vi "Vision Processing.vi"(7 "CameraDevRef":T1) -> ()   [LabVIEW 2011]
doc: "This VI runs in parallel to other tasks. It gets images from the camera, processes them for color or shape and use that information to affect robot behavior."
uses:
  <vilib>/Rock Robotics/WPI/Camera/WPI_CameraDevRef.ctl
  Robot Global Data.vi
  <vilib>/vision/NI_Vision_Development_Module.lvlib
panel:
  in  "Case to run":dbl=2.0
  in  "Manual Overide":bool
  out "Target Distance":dbl
  out "Target Y Coord":dbl
  out "Distance Array":dbl[](array[numeric])
  in  "Scaler":dbl=0.85
  in  "Enable Imaging on Screen":bool
  out "Target X Coord":dbl
  in  "Lower Speed Limit":dbl=0.05
  out "Turret Rotation":dbl
  out "Number of Rectangles Visible":dbl
  out "Y Position Array":dbl[](array[numeric])
  out "X Position Array":dbl[](array[numeric])
  out "Array":T2(array[cluster])
  in  "Score Limits":T3={"Rect Coverage"=76.0, "Aspect Ratio"=40.0, "X Edge Strength"=40.0, "Y Edge Strength"=60.0}
  out "Processed Image":T4(plugin-control)
  out "Original Image":T4(plugin-control)
  in  "Annotate":bool=TRUE
  in  "Particle Count Limit":i32=10
  in  "Area Size Limit":i32=444
  in  "Range":cluster{"Lower value":sgl, "Upper value":sgl}={"Lower value"=120.0, "Upper value"=255.0}
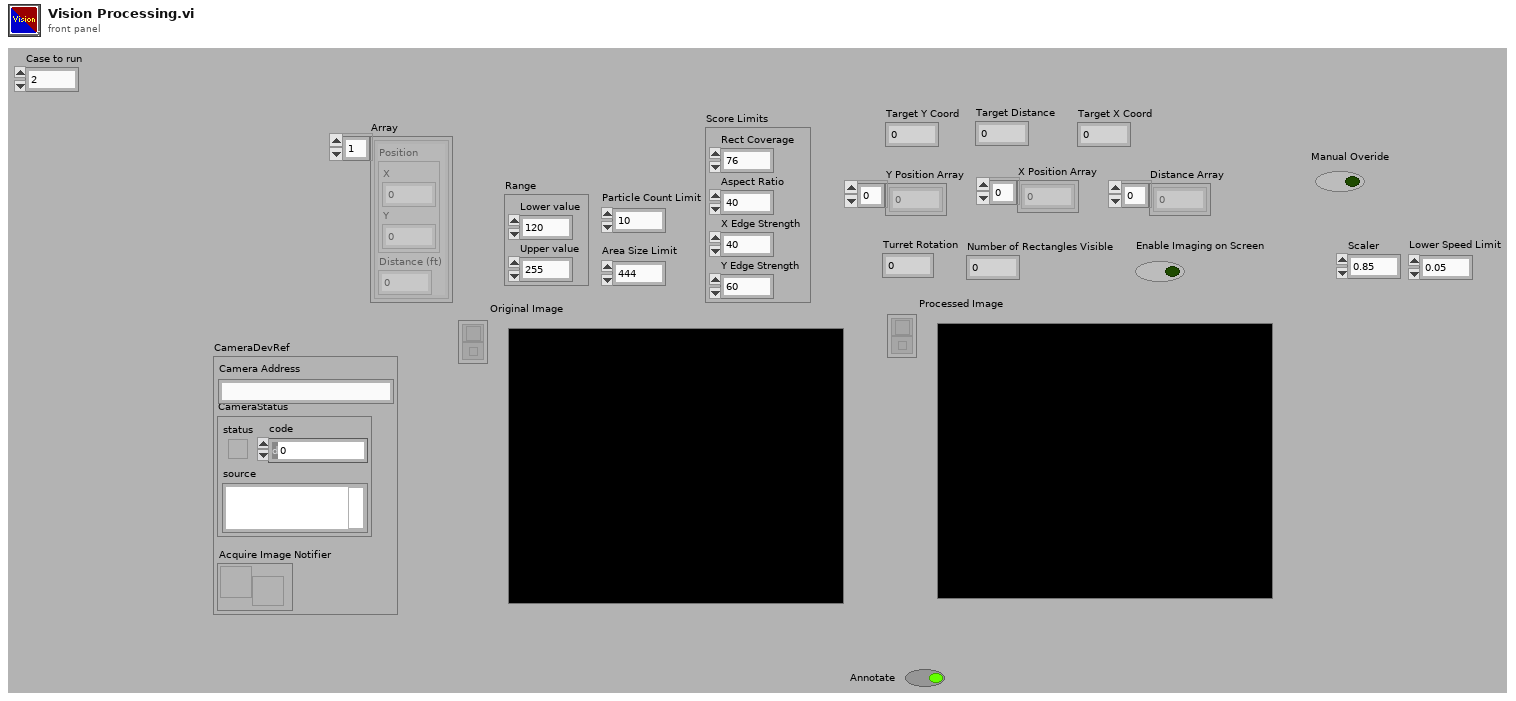
[diagram p1: front panel]
types:
  T1 = typedef "WPI_CameraDevRef.ctl" = cluster{"Camera Address":string, "CameraStatus":errorcluster, "Acquire Image Notifier":refnum<notifier>}
  T2 = cluster{"Position":cluster{"X":dbl, "Y":dbl}, "Distance (ft)":dbl}[]
  T3 = cluster{"Rect Coverage":dbl, "Aspect Ratio":dbl, "X Edge Strength":dbl, "Y Edge Strength":dbl}
  T4 = typedef "IMAQ Image.ctl" = refnum<image>
  T5 = typedef "Image Type" = u32
  T6 = cluster{cluster{"Left":dbl, "Top":dbl, "Right":dbl, "Bottom":dbl}, dbl[]}[]
  T7 = cluster{"Left":dbl, "Top":dbl, "Right":dbl, "Bottom":dbl}
  T8 = cluster{"Target Center (-1 to 1)":cluster{"X":dbl, "Y":dbl}, "Distance (ft)":dbl}
  T9 = cluster{"Target Center (-1 to 1)":cluster{"X":dbl, "Y":dbl}, "Distance (ft)":dbl}[]
  T10 = cluster{"Axis 1":dbl, "Axis 2":dbl, "Axis 3":dbl, "Axis 4":dbl, "Axis 5":dbl, "Axis 6":dbl, "Button 1":bool, "Button 2":bool, "Button 3":bool, "Button 4":bool, "Button 5":bool, "Button 6":bool, "Button 7":bool, "Button 8":bool, "Button 9":bool, "Button 10":bool, "Button 11":bool, "Button 12":bool}
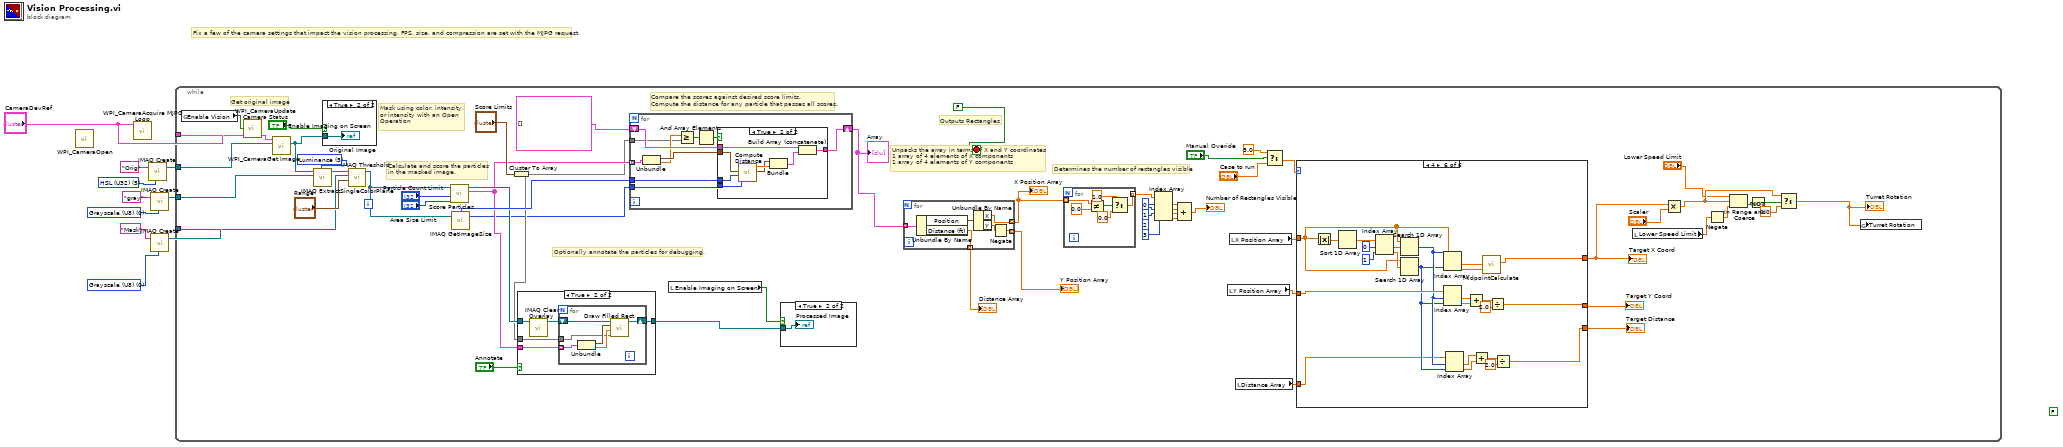
[diagram p0: block diagram]
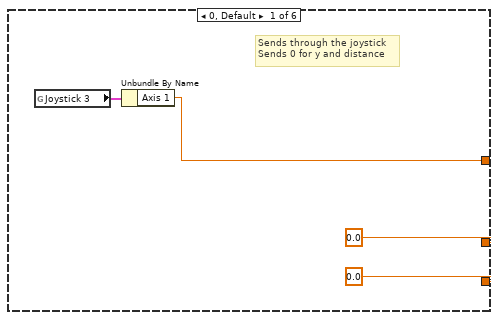
[diagram p4: hidden frame]
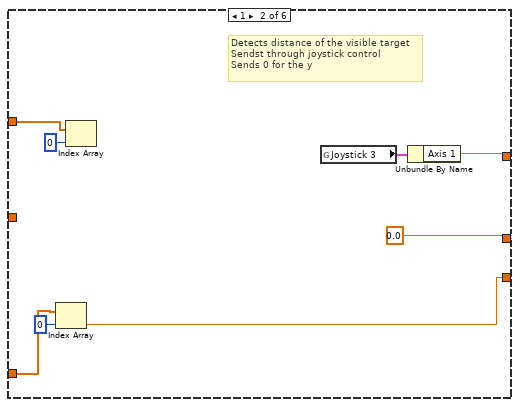
[diagram p5: hidden frame]
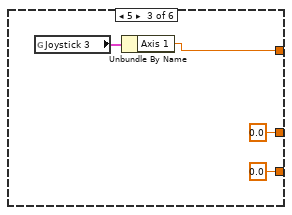
[diagram p6: hidden frame]
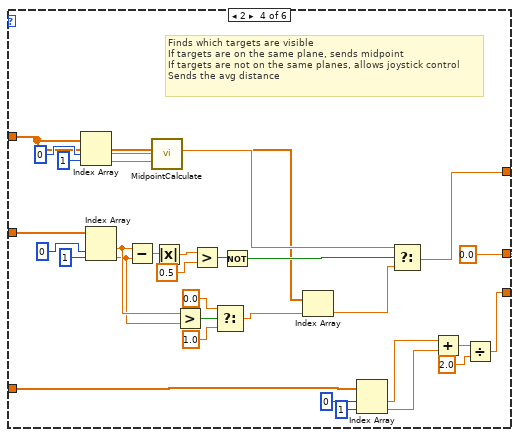
[diagram p7: hidden frame]
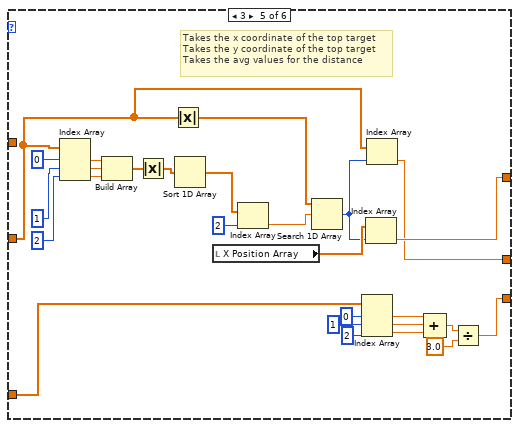
[diagram p8: hidden frame]
diagram:
  w3 = T5 5 items=["Grayscale (U8)", "Grayscale (I16)", "Grayscale (SGL)", "Complex (CSG)", "RGB (U32)", "HSL (U32)", "RGB (U64)", "Grayscale (U16)"] ("Image Type")
  (unwired) FALSE
  w6 = T5 0 items=["Grayscale (U8)", "Grayscale (I16)", "Grayscale (SGL)", "Complex (CSG)", "RGB (U32)", "HSL (U32)", "RGB (U64)", "Grayscale (U16)"] ("Image Type")
  w10 = T5 0 items=["Grayscale (U8)", "Grayscale (I16)", "Grayscale (SGL)", "Complex (CSG)", "RGB (U32)", "HSL (U32)", "RGB (U64)", "Grayscale (U16)"] ("Image Type")
  # "Fix a few of the camera settings that impact the vision processing. FPS, size, and compression are set with the MJPG request."
  n1 = call <vilib>:"WPI_CameraOpen.vi"() -> ()  [unwired: 10 in, 2 out]
  n2 = call <vilib>:"WPI_CameraAcquire MJPG Loop.vi"("CameraDevRef"="CameraDevRef") -> ()  [unwired: 11 in]
  n3 = call "IMAQ Create"("Image Name"="Orig", "Image Type"=w3) -> ("New Image"=w2:T4)  [unwired: 2 in, 2 out]
  n4 = call "IMAQ Create"("Image Name"="gray", "Image Type"=w10) -> ("New Image"=w8:T4)  [unwired: 2 in, 2 out]
  n5 = call "IMAQ Create"("Image Name"="Mask", "Image Type"=w6) -> ("New Image"=w5:T4)  [unwired: 2 in, 2 out]
  n6 = while {
    tunnel: w8 -> [w53]
    tunnel: w5 -> [w54]
    tunnel: w2 -> [w37]
    tunnel: "CameraDevRef" -> [w35]
    stop <- FALSE stop-if-true
    w57 = 5 items=["Red", "Green", "Blue", "Hue", "Saturation", "Luminance", "Value", "Intensity"] ("Color Plane")
    # "Determines the number of rectangles visible"
    # "Unpacks the array in terms of X and Y coordinates\n1 array of 4 elements of X components\n1 array of 4 elements of Y components"
    # "Outputs Rectangles"
    # "Optionally annotate the particles for debugging."
    # "Compare the scores against desired score limits.\nCompute the distance for any particle that passes all scores."
    # "Calculate and score the particles\nin the masked image."
    # "Mask using color, intensity,\nor intensity with an Open\nOperation"
    # "Get original image"
    n7 = global read "Robot Global Data.vi" "Enable Vision"() -> (w34:bool)
    n8 = call <vilib>:"WPI_CameraUpdate Camera Status.vi"("CameraDevRef In"=w35, "Enable Vision"=w34) -> ("CameraDevRef Out"=w36:T1)  [unwired: 3 in]
    n9 = call <vilib>:"WPI_CameraGet Image.vi"("Image"=w37, "CameraDevRef"=w36) -> ("Image Out"=w33:T4)  [unwired: 7 in, 2 out]
    n10 = call "IMAQ ExtractSingleColorPlane"("Color Plane"=w57, "Image Dst"=w53, "Image Src"=w33) -> ("Image Dst Out"=w55:T4)  [unwired: 1 in, 7 out]
    n11 = case shown="True" "Enable Imaging on Screen" {
      tunnel: w33 -> [_ w70]
      frame False {
      }
      frame True {
        "Original Image" <- w70
      }
    }
    n12 = call "IMAQ Threshold"("Range"="Range", "Image Dst"=w54, "Image Src"=w55) -> ("Image Dst Out"=w52:T4)  [unwired: 3 in, 5 out]
    n13 = call "Score Particles.vi"("Area Size Limit"="Area Size Limit", "Particle Count Limit"="Particle Count Limit", "Image Refnum in"=w52) -> ("Scored Particle Info"=w64:T6, "Image Refnum out"=w67:T4)  [unwired: 7 in]
    n14 = call "IMAQ GetImageSize"("Image"=w52) -> ("Y Resolution"=w58:i32, "X Resolution"=w68:i32)  [unwired: 3 in, 1 out]
    n15 = Cluster To Array(cluster="Score Limits") -> (array=w62:dbl[])
    n16 = case shown="True" "Annotate" {
      tunnel: w67 -> [w181 w186]
      tunnel: [w181 w185] -> w65
      tunnel: w64 -> [_ w183]
      tunnel: w62 -> [_ w182]
      frame False {
      }
      frame True {
        n17 = call "IMAQ Clear Overlay"("Image"=w186) -> ("Image Out"=w184:T4)  [unwired: 2 in, 8 out]
        n18 = for {
          shift-right: [w191] -> w185
          shift-left: w184 -> [w192]
          tunnel: w183 -> [w188] mode=indexing
          tunnel: w182 -> [w187]
          n19 = Unbundle(w188) -> (w189:T7, w190:dbl[])
          n20 = call "Draw Filled Rect.vi"("Limits"=w187, "Scores"=w190, "Bounding Box"=w189, "image in"=w192) -> ("image out"=w191:T4)  [unwired: 7 in]
        }
      }
    }
    n21 = for {
      shift-right: [w201] -> w38
      shift-left: T2 [] -> [w202]
      tunnel: w68 -> [w200]
      tunnel: w64 -> [w198] mode=indexing
      tunnel: w62 -> [w194]
      tunnel: w58 -> [w193]
      n22 = Unbundle(w198) -> (w199:T7, w195:dbl[])
      n23 = Greater Or Equal?(x=w195, y=w194) -> (x >= y?=w197:bool[])
      n24 = And Array Elements(Boolean array=w197) -> (logical AND=w196:bool)
      n25 = case shown="True" w196 {
        tunnel: w202 -> [w203 w211]
        tunnel: [w203 w210] -> w201
        tunnel: w199 -> [_ w206]
        tunnel: w200 -> [_ w208]
        tunnel: w193 -> [_ w204]
        frame False {
        }
        frame True {
          n26 = call "Compute Distance.vi"("Y Image Resolution"=w204, "X Image Resolution"=w208, "Bounding Box"=w206) -> ("Target Center (-1 to 1)"=w205:cluster{"X":dbl, "Y":dbl}, "Distance (ft)"=w207:dbl)  [unwired: 7 in]
          n27 = Bundle("Target Center (-1 to 1)"=w205, "Distance (ft)"=w207) -> (w209:T8)  [unwired: 1 in]
          n28 = Build Array (concatenate)(w211, w209) -> (w210:T9)
        }
      }
    }
    "Array" <- w38
    n29 = local read "Enable Imaging on Screen"() -> (w31:bool)
    n30 = case shown="True" w31 {
      tunnel: w65 -> [_ w69]
      frame False {
      }
      frame True {
        "Processed Image" <- w69
      }
    }
    n31 = for {
      tunnel: [w178] -> w50 mode=indexing
      tunnel: [w179] -> w40 mode=indexing
      tunnel: w38 -> [w176] mode=indexing
      tunnel: [w175] -> w23 mode=indexing
      n32 = Unbundle By Name(w176) -> ("Position"=w180:cluster{"X":dbl, "Y":dbl}, "Distance (ft)"=w175:dbl)
      n33 = Unbundle By Name(w180) -> ("X"=w179:dbl, "Y"=w177:dbl)
      n34 = Negate(x=w177) -> (-x=w178:dbl)
    }
    "X Position Array" <- w40
    "Y Position Array" <- w50
    "Distance Array" <- w23
    n35 = for {
      tunnel: w40 -> [w75] mode=indexing
      tunnel: [w71] -> w41 mode=indexing
      n36 = Not Equal?(x=w75, y=0.0) -> (x != y?=w74:bool)
      n37 = Select(t=1.0, s=w74, f=0.0) -> (s? t:f=w71:dbl)
    }
    n38 = Index Array(array=w41, index #1=0 ("index"), index #2=1 ("index"), index #3=2 ("index"), index #4=3 ("index")) -> (element #1=w43:dbl, element #2=w42:dbl, element #3=w44:dbl, element #4=w45:dbl)
    n39 = Compound Arithmetic op=ADD(w43, w42, w44, w45) -> (→"Number of Rectangles Visible":dbl)
    n40 = local read "Y Position Array"() -> (w19:dbl[])
    n41 = local read "X Position Array"() -> (w39:dbl[])
    n42 = local read "Distance Array"() -> (w18:dbl[])
    n43 = Select(t=5.0, s="Manual Overide", f="Case to run") -> (s? t:f=w14:dbl)
    n44 = case shown="4" w14 {
      tunnel: w39 -> [_ w83 _ w94 _ w168]
      tunnel: [w79 w81 w91 w112 w137 w165] -> w20
      tunnel: [0.0 ("X") 0.0 ("X") 0.0 ("X") 0.0 ("X") w136 w159] -> w22
      tunnel: [0.0 ("X") w86 0.0 ("X") w105 w126 w151] -> w21
      tunnel: w19 -> [_ _ _ w121 w124 w164]
      tunnel: w18 -> [_ w88 _ w104 w125 w156]
      frame 0, Default {
        # "Sends through the joystick\nSends 0 for y and distance"
        n45 = global read "Robot Global Data.vi" "Joystick 3"() -> (w80:T10)
        n46 = Unbundle By Name(w80) -> ("Axis 1"=w79:dbl)
      }
      frame 1 {
        # "Detects distance of the visible target\nSendst through joystick control\nSends 0 for the y"
        n47 = Index Array(array=w88, index=0) -> (element=w86:dbl)
        n48 = Index Array(array=w83, index=0) -> ()  [unwired: 1 out]
        n49 = global read "Robot Global Data.vi" "Joystick 3"() -> (w82:T10)
        n50 = Unbundle By Name(w82) -> ("Axis 1"=w81:dbl)
      }
      frame 5 {
        n51 = global read "Robot Global Data.vi" "Joystick 3"() -> (w92:T10)
        n52 = Unbundle By Name(w92) -> ("Axis 1"=w91:dbl)
      }
      frame 2 {
        # "Finds which targets are visible\nIf targets are on the same plane, sends midpoint\nIf targets are not on the same planes, allows joystick control\nSends the avg distance"
        n53 = Index Array(array=w94, index #1=0 ("index"), index #2=1 ("index")) -> (element #1=w110:dbl, element #2=w109:dbl)
        n54 = Index Array(array=w121, index #1=0 ("index"), index #2=1 ("index")) -> (element #1=w100:dbl, element #2=w99:dbl)
        n55 = Subtract(x=w100, y=w99) -> (x-y=w118:dbl)
        n56 = call "MidpointCalculate.vi"("X2"=w109, "X1"=w110) -> ("Midpoint"=w113:dbl)  [unwired: 9 in]
        n57 = Absolute Value(x=w118) -> (abs(x)=w117:dbl)
        n58 = Greater?(x=w100, y=w99) -> (0:w98:bool)
        n59 = Greater?(x=w117, y=0.5) -> (0:w114:bool)
        n60 = Select(t=0.0, s=w98, f=1.0) -> (s? t:f=w95:dbl)
        n61 = Not(x=w114) -> (.not. x?=w115:bool)
        n62 = Index Array(array=w94, index=w95) -> (element=w93:dbl)
        n63 = Index Array(array=w104, index #1=0 ("index"), index #2=1 ("index")) -> (element #1=w103:dbl, element #2=w102:dbl)
        n64 = Select(t=w113, s=w115, f=w93) -> (s? t:f=w112:dbl)
        n65 = Add(x=w103, y=w102) -> (x+y=w108:dbl)
        n66 = Divide(x=w108, y=2.0) -> (x/y=w105:dbl)
      }
      frame 3 {
        # "Takes the x coordinate of the top target\nTakes the y coordinate of the top target\nTakes the avg values for the distance"
        n67 = Index Array(array=w124, index #1=0 ("index"), index #2=1 ("index"), index #3=2 ("index")) -> (element #1=w147:dbl, element #2=w146:dbl, element #3=w145:dbl)
        n68 = Build Array(w147, w146, w145) -> (w144:dbl[])
        n69 = Absolute Value(x=w144) -> (abs(x)=w141:dbl[])
        n70 = Absolute Value(x=w124) -> (abs(x)=w142:dbl[])
        n71 = Sort 1D Array(array=w141) -> (sorted array=w140:dbl[])
        n72 = local read "X Position Array"() -> (w138:dbl[])
        n73 = Index Array(array=w140, index=2) -> (element=w139:dbl)
        n74 = Search 1D Array(1D array=w142, element=w139) -> (index of element=w135:i32)  [unwired: 1 in]
        n75 = Index Array(array=w125, index #1=0 ("index"), index #2=1 ("index"), index #3=2 ("index")) -> (element #1=w131:dbl, element #2=w130:dbl, element #3=w129:dbl)
        n76 = Index Array(array=w138, index=w135) -> (element=w137:dbl)
        n77 = Index Array(array=w124, index=w135) -> (element=w136:dbl)
        n78 = Compound Arithmetic op=ADD(w131, w130, w129) -> (w128:dbl)
        n79 = Divide(x=w128, y=3.0) -> (x/y=w126:dbl)
      }
      frame 4 {
        n80 = Absolute Value(x=w168) -> (abs(x)=w174:dbl[])
        n81 = Sort 1D Array(array=w174) -> (sorted array=w173:dbl[])
        n82 = Index Array(array=w173, index #1=0 ("index"), index #2=1 ("index")) -> (element #1=w169:dbl, element #2=w170:dbl)
        n83 = Search 1D Array(1D array=w168, element=w169) -> (index of element=w158:i32)  [unwired: 1 in]
        n84 = Search 1D Array(1D array=w168, element=w170) -> (index of element=w157:i32)  [unwired: 1 in]
        n85 = Index Array(array=w168, index #1=w158, index #2=w157) -> (element #1=w167:dbl, element #2=w166:dbl)
        n86 = Index Array(array=w164, index #1=w158, index #2=w157) -> (element #1=w162:dbl, element #2=w163:dbl)
        n87 = Index Array(array=w156, index #1=w158, index #2=w157) -> (element #1=w153:dbl, element #2=w152:dbl)
        n88 = Add(x=w162, y=w163) -> (x+y=w161:dbl)
        n89 = Add(x=w153, y=w152) -> (x+y=w154:dbl)
        n90 = call "MidpointCalculate.vi"("X2"=w166, "X1"=w167) -> ("Midpoint"=w165:dbl)  [unwired: 9 in]
        n91 = Divide(x=w161, y=2.0) -> (x/y=w159:dbl)
        n92 = Divide(x=w154, y=2.0) -> (x/y=w151:dbl)
      }
    }
    "Target Y Coord" <- w22
    "Target Distance" <- w21
    "Target X Coord" <- w20
    n93 = local read "Lower Speed Limit"() -> (w29:dbl)
    n94 = Multiply(x=w20, y="Scaler") -> (x*y=w24:dbl)
    n95 = Negate(x=w29) -> (-x=w28:dbl)
    n96 = In Range and Coerce(upper limit="Lower Speed Limit", x=w24, lower limit=w28) -> (In Range?=w27:bool)  [unwired: 1 out]
    n97 = Not(x=w27) -> (.not. x?=w26:bool)
    n98 = Select(t=w24, s=w26, f=0.0) -> (s? t:f=w12:dbl)
    "Turret Rotation" <- w12
    n99 = global write "Robot Global Data.vi" "Turret Rotation"(w12) -> ()
  }
